vi "Compare Model Info - SysDef vs Model DLL.vi"(0 "System Definition Filepath (.nivssdf)":path, 11 "Error (in)":errorcluster) -> (15 "Error (out)":errorcluster)   [LabVIEW 2016]
panel:
  out "Signals Added":string[](array[string])
  out "Signals Removed":string[](array[string])
  out "SysDef Signals":string[](array[string])
  out "DLL Signals":string[](array[string])
  out "Parameters Added":string[](array[string])
  out "Parameters Removed":string[](array[string])
  out "SysDef Parameters":string[](array[string])
  out "DLL Parameters":string[](array[string])
  out "Outports Added":string[](array[string])
  out "Outports Removed":string[](array[string])
  out "SysDef Outports":string[](array[string])
  out "DLL Outports":string[](array[string])
  out "Inports Added":string[](array[string])
  out "Inports Removed":string[](array[string])
  out "SysDef Inports":string[](array[string])
  out "DLL Inports":string[](array[string])
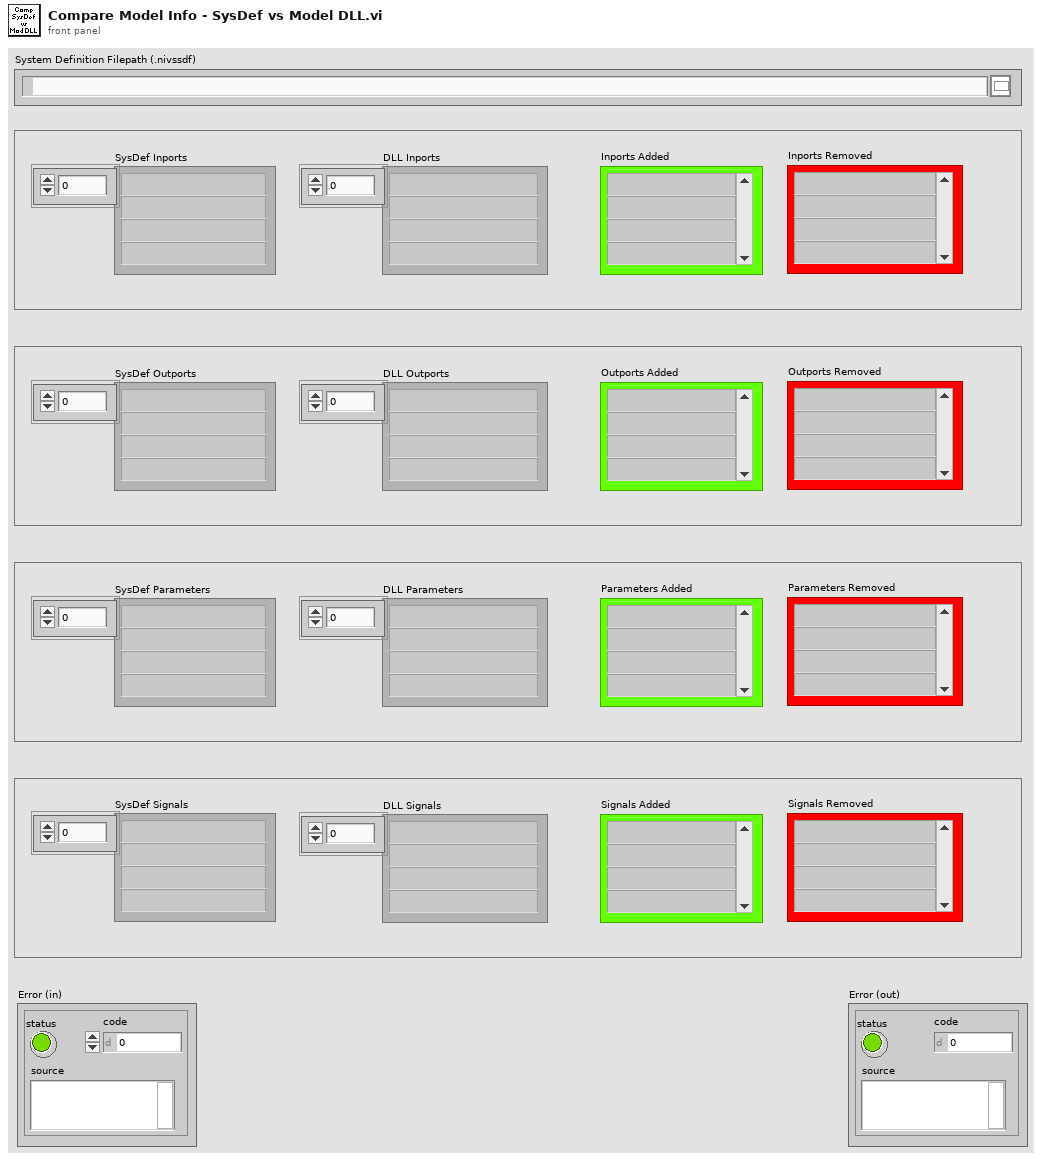
[diagram p1: front panel]
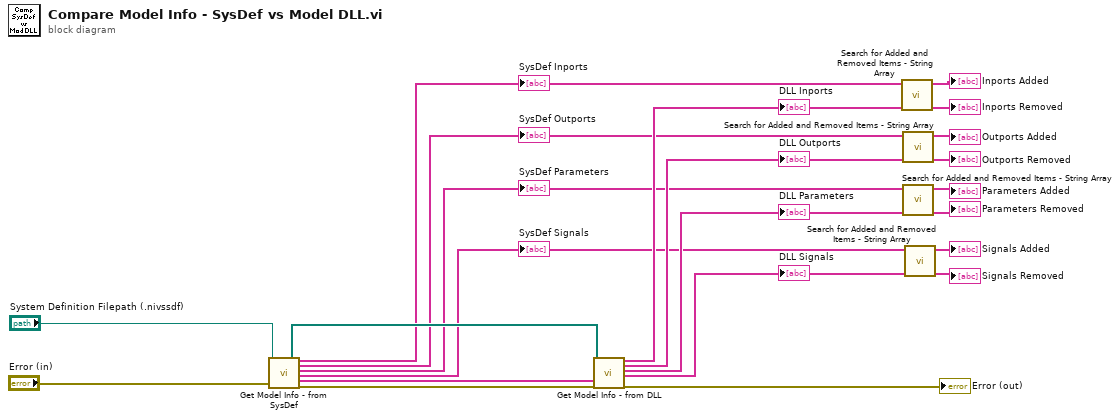
[diagram p0: block diagram]
diagram:
  n1 = call "Get Model Info - from SysDef.vi"("System Definition Filepath (.nivssdf)"="System Definition Filepath (.nivssdf)", "Error (in)"="Error (in)") -> ("Model Filepaths"=w18:path[], "SysDef Inports"=w15:string[], "SysDef Outports"=w12:string[], "SysDef Parameters"=w10:string[], "SysDef Signals"=w5:string[], "Models"=w17:string[], "Error (out)"=w20:errorcluster)  [unwired: 11 in]
  "SysDef Inports" <- w15
  "SysDef Outports" <- w12
  "SysDef Parameters" <- w10
  "SysDef Signals" <- w5
  n2 = call "Get Model Info - from DLL.vi"("Model Filepaths"=w18, "Models"=w17, "Error (in)"=w20) -> ("DLL Inports"=w16:string[], "DLL Outports"=w11:string[], "DLL Parameters"=w9:string[], "DLL Signals"=w6:string[], "Error (out)"=→"Error (out)":errorcluster)  [unwired: 12 in]
  "DLL Inports" <- w16
  "DLL Outports" <- w11
  "DLL Parameters" <- w9
  "DLL Signals" <- w6
  n3 = call "Search for Added and Removed Items - String Array.vi"("Model"=w16, "SysDef"=w15) -> ("Model Items Removed"=→"Inports Removed":string[], "Model Items Added"=→"Inports Added":string[])  [unwired: 8 in]
  n4 = call "Search for Added and Removed Items - String Array.vi"("Model"=w11, "SysDef"=w12) -> ("Model Items Removed"=→"Outports Removed":string[], "Model Items Added"=→"Outports Added":string[])  [unwired: 8 in]
  n5 = call "Search for Added and Removed Items - String Array.vi"("Model"=w9, "SysDef"=w10) -> ("Model Items Removed"=→"Parameters Removed":string[], "Model Items Added"=→"Parameters Added":string[])  [unwired: 8 in]
  n6 = call "Search for Added and Removed Items - String Array.vi"("Model"=w6, "SysDef"=w5) -> ("Model Items Removed"=→"Signals Removed":string[], "Model Items Added"=→"Signals Added":string[])  [unwired: 8 in]
